vi "hw2p2_hickey.vi"() -> ()   [LabVIEW 2014]
panel:
  out "Waveform Chart":dbl(graph)
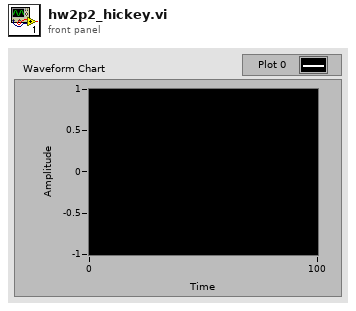
[diagram p1: front panel]
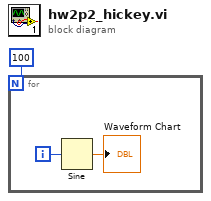
[diagram p0: block diagram]
diagram:
  n1 = for {
    N: 100 -> [_]
    i -> [w3]
    n2 = Sine(x=w3) -> (sin(x)=→"Waveform Chart":dbl)
  }
